vi "Uncompress SEQ line.vi"(4 "error in":errorcluster, 6 "SEQ file refnum":refnum<file>) -> (0 "error out":errorcluster, 2 "Pixel Array":u8[](array[numeric]))   [LabVIEW 2016]
doc: "// *******************************************************************\nBYTE *unCompress( int length, BYTE *buffer )\n{\n BYTE *s,*d, dif;\n WORD pixel;\n\n s = buffer;\n d = full; /* Set up buffer pointers */\n *d++ = *s++; /* Get first pixel */\n length--; /* and adjust counter */\n while (length-- > 0) /* While not EOL */\n {\n pixel = *(WORD *)s++; /* Fetch TWO bytes! */\n // Process the even nibble.\n if ((pixel & 0x0f) == 0x0f)\n { // A nibble of 15 indicates overflow;Next byte contains\n // a new pixel. This byte is on an odd nibble boundary, and mask.\n *d++ = (BYTE)((pixel >> 4) & 0xff); /* Next whole pixel */\n pixel = (WORD)*s++; /* Read next byte */\n length--; /* and adjust counter */\n }\n else\n { // Regular signed nibble difference\n dif = (BYTE)(pixel & 0x0F);\n if (pixel & 0x08)\n *d = (BYTE) (*(d-1) - (dif - 7));\n else\n *d = (BYTE) (*(d-1) + dif);\n d++;\n }\n // Now process the odd nibble.\n if ((pixel & 0xf0) == 0xf0)\n { // A nibble of 15 indicates overflow; Next byte contains a new\n // pixel. This byte is on a byte boundary, so simply fetch it.\n *d++ = *s++; /* Next pixel */\n length--; /* and adjust counter */\n }\n else\n { // Regular signed nibble difference\n dif = (BYTE)((pixel & 0xF0) >>4);\n if (pixel & 0x80)\n *d = (BYTE) (*(d-1) - (dif -7));\n else\n *d = (BYTE) (*(d-1) + dif);\n d++; /* Increment destination */\n }\n }\n return(full);\n}"
panel:
  out "#bytes in\ncompressed\nline":u16(graph)
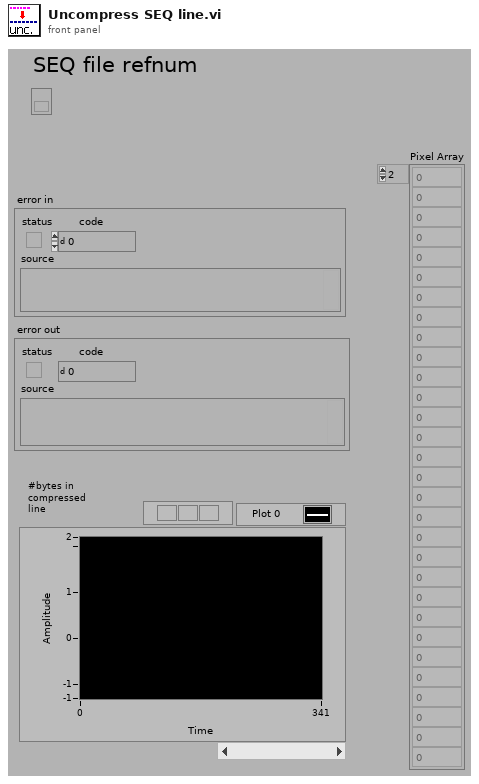
[diagram p1: front panel]
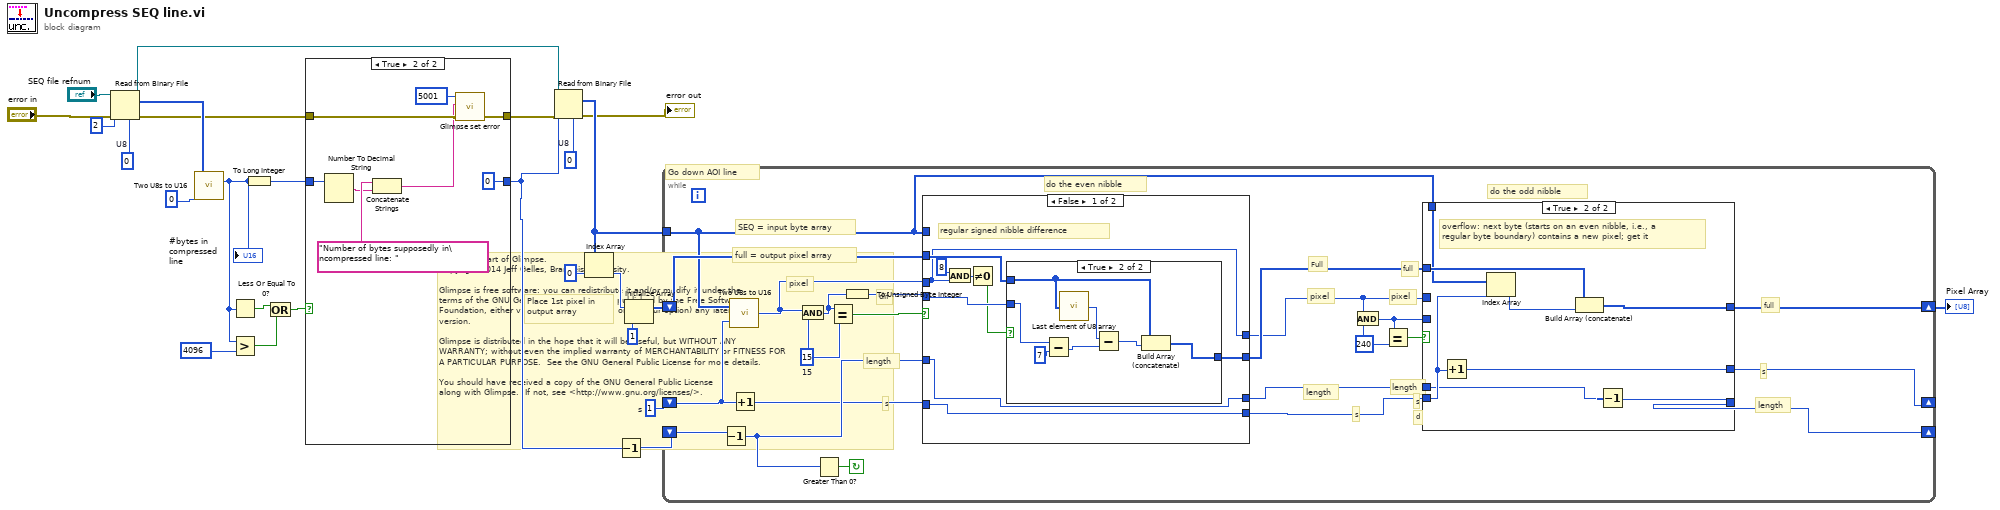
[diagram p0: block diagram]
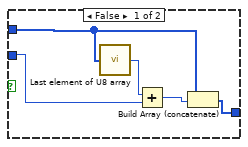
[diagram p3: hidden frame]
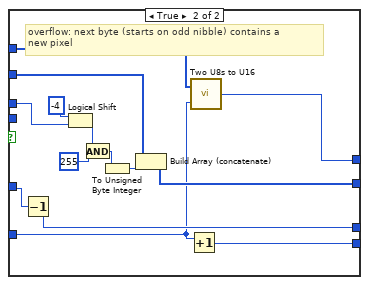
[diagram p4: hidden frame]
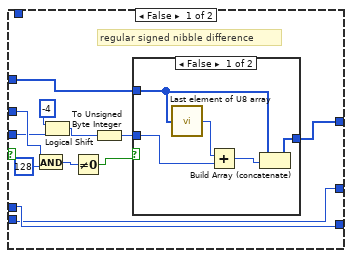
[diagram p5: hidden frame]
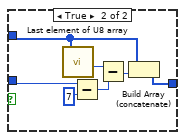
[diagram p6: hidden frame]
diagram:
  w15 = 1  # s
  w18 = u8 0  # U8
  w23 = u8 0  # U8
  # "This file is part of Glimpse. \nCopyright 2014 Jeff Gelles, Brandeis University.    \n\nGlimpse is free software: you can redistribute it and/or modify it under the \nterms of the GNU General Public License as published by the Free Software \nFoundation, either version 3 of the License, or (at your option) any later \nversion.\n\nGlimpse is distributed in the hope that it will be useful, but WITHOUT ANY \nWARRANTY; without even the implied warranty of MERCHANTABILITY or FITNESS FOR \nA PARTICULAR PURPOSE.  See the GNU General Public License for more details.\n\nYou should have received a copy of the GNU General Public License\nalong with Glimpse.  If not, see <http://www.gnu.org/licenses/>."
  # "Place 1st pixel in\noutput array"
  # "Go down AOI line"
  n1 = Read from Binary File(5:w23, 8:"error in", 10:2 ("count"), 11:"SEQ file refnum") -> (0:w2:errorcluster, 2:w19:u8[], 3:w17:refnum<file>)  [unwired: 3 out]
  n2 = call "Two U8s to U16.vi"("Index of first byte"=0 ("index"), "Byte array"=w19) -> ("Output word"=w6:u16)
  "#bytes in\ncompressed\nline" <- w6
  n3 = Less Or Equal To 0?(x=w6) -> (x <= 0?=w9:bool)
  n4 = Greater?(x=w6, y=u16 4096) -> (0:w5:bool)
  n5 = To Long Integer(number=w6) -> (32bit integer=w4:i32)
  n6 = Or(x=w9, y=w5) -> (x .or. y?=w8:bool)
  n7 = case shown="True" w8 {
    tunnel: w4 -> [w28 w32]
    tunnel: [w28 0] -> w3
    tunnel: w2 -> [w27 w34]
    tunnel: [w27 w35] -> w1
    frame False {
    }
    frame True {
      n8 = Number To Decimal String(number=w32) -> (decimal integer string=w30:string)  [unwired: 1 out]
      n9 = Concatenate Strings("Number of bytes supposedly in\ncompressed line: " ("string"), w30) -> (w29:string)
      n10 = call "Glimpse set error.vi"("code"=5001, "Additional information"=w29, "error in"=w34) -> ("error out"=w35:errorcluster)  [unwired: 5 out]
    }
  }
  n11 = Read from Binary File(5:w18, 8:w1, 10:w3, 11:w17) -> (0:→"error out":errorcluster, 2:w16:u8[])  [unwired: 4 out]
  n12 = Index Array(array=w16, index=0) -> (element=w13:u8)
  n13 = Decrement(x=w3) -> (x-1=w26:i32)
  n14 = Initialize Array(w13, 1) -> (w12:u8[])
  n15 = while {
    tunnel: w16 -> [w37]
    shift-left: w12 -> [w52]
    shift-right: [w40] -> w11
    shift-left: w26 -> [w55]
    shift-right: [w38] -> _
    shift-left: w15 -> [w50]
    shift-right: [w39] -> _
    stop <- w53 continue-if-true
    w45 = u8 240 ("15")
    w58 = u8 15  # 15
    # "do the even nibble"
    # "s"
    # "s"
    # "full"
    # "pixel"
    # "d"
    # "s"
    # "length"
    # "full"
    # "length"
    # "do the odd nibble"
    # "pixel"
    # "SEQ = input byte array"
    # "full = output pixel array"
    # "s"
    # "length"
    # "pixel"
    # "length"
    # "Full"
    # "dif"
    n16 = Decrement(x=w55) -> (x-1=w54:i32)
    n17 = call "Two U8s to U16.vi"("Index of first byte"=w50, "Byte array"=w37) -> ("Output word"=w49:u16)
    n18 = Increment(x=w50) -> (x+1=w51:i32)
    n19 = And(x=w49, y=w58) -> (x .and. y?=w56:u16)
    n20 = Greater Than 0?(x=w54) -> (x > 0?=w53:bool)
    n21 = Equal?(x=w56, y=w58) -> (x = y?=w57:bool)
    n22 = To Unsigned Byte Integer(number=w56) -> (unsigned 8bit integer=w48:u8)
    n23 = case shown="False" w57 {
      tunnel: w51 -> [w63 w80]
      tunnel: [w63 w93] -> w41
      tunnel: w49 -> [w59 w85]
      tunnel: w48 -> [w67 _]
      tunnel: [w62 w87] -> w44
      tunnel: w54 -> [w61 w92]
      tunnel: [w61 w91] -> w42
      tunnel: w52 -> [w60 w86]
      tunnel: [w59 w82] -> w43
      tunnel: w37 -> [_ w81]
      frame False {
        # "regular signed nibble difference"
        n24 = And(x=u8 8 ("15"), y=w59) -> (x .and. y?=w66:u16)
        n25 = Not Equal To 0?(x=w66) -> (x != 0?=w64:bool)
        n26 = case shown="True" w64 {
          tunnel: w67 -> [w70 w79]
          tunnel: w60 -> [w69 w75]
          tunnel: [w68 w77] -> w62
          frame False {
            n27 = call "Last element of U8 array.vi"("Array"=w69) -> ("Last element"=w71:u8)
            n28 = Add(x=w71, y=w70) -> (x+y=w72:u8)
            n29 = Build Array (concatenate)(w69, w72) -> (w68:u8[])
          }
          frame True {
            n30 = Subtract(x=w79, y=u8 7) -> (x-y=w74:u8)
            n31 = call "Last element of U8 array.vi"("Array"=w75) -> ("Last element"=w76:u8)
            n32 = Subtract(x=w76, y=w74) -> (x-y=w73:u8)
            n33 = Build Array (concatenate)(w75, w73) -> (w77:u8[])
          }
        }
      }
      frame True {
        # "overflow: next byte (starts on odd nibble) contains a \nnew pixel"
        n34 = Decrement(x=w92) -> (x-1=w91:i32)
        n35 = Logical Shift(y=i16 -4, x=w85) -> (x << y=w89:u16)
        n36 = And(x=w89, y=u8 255) -> (x .and. y?=w84:u16)
        n37 = To Unsigned Byte Integer(number=w84) -> (unsigned 8bit integer=w83:u8)
        n38 = Build Array (concatenate)(w86, w83) -> (w87:u8[])
        n39 = Increment(x=w80) -> (x+1=w93:i32)
        n40 = call "Two U8s to U16.vi"("Index of first byte"=w80, "Byte array"=w81) -> ("Output word"=w82:u16)
      }
    }
    n41 = And(x=w43, y=w45) -> (x .and. y?=w47:u16)
    n42 = Equal?(x=w47, y=w45) -> (x = y?=w46:bool)
    n43 = case shown="True" w46 {
      tunnel: w41 -> [w98 w124]
      tunnel: w44 -> [w99 w119]
      tunnel: [w101 w125] -> w40
      tunnel: [w105 w122] -> w38
      tunnel: w42 -> [w105 w121]
      tunnel: w43 -> [w100 _]
      tunnel: [w98 w123] -> w39
      tunnel: w47 -> [w97 _]
      tunnel: w37 -> [_ w118]
      frame False {
        # "regular signed nibble difference"
        n44 = And(x=w100, y=u8 128) -> (x .and. y?=w95:u16)
        n45 = Logical Shift(y=i16 -4, x=w97) -> (x << y=w102:u16)
        n46 = Not Equal To 0?(x=w95) -> (x != 0?=w94:bool)
        n47 = To Unsigned Byte Integer(number=w102) -> (unsigned 8bit integer=w96:u8)
        n48 = case shown="False" w94 {
          tunnel: w96 -> [w106 w117]
          tunnel: [w108 w112] -> w101
          tunnel: w99 -> [w107 w113]
          frame False {
            n49 = call "Last element of U8 array.vi"("Array"=w107) -> ("Last element"=w110:u8)
            n50 = Add(x=w110, y=w106) -> (x+y=w109:u8)
            n51 = Build Array (concatenate)(w107, w109) -> (w108:u8[])
          }
          frame True {
            n52 = call "Last element of U8 array.vi"("Array"=w113) -> ("Last element"=w115:u8)
            n53 = Subtract(x=w117, y=u8 7) -> (x-y=w114:u8)
            n54 = Subtract(x=w115, y=w114) -> (x-y=w111:u8)
            n55 = Build Array (concatenate)(w113, w111) -> (w112:u8[])
          }
        }
      }
      frame True {
        # "overflow: next byte (starts on an even nibble, i.e., a\nregular byte boundary) contains a new pixel; get it"
        n56 = Increment(x=w124) -> (x+1=w123:i32)
        n57 = Index Array(array=w118, index=w124) -> (element=w120:u8)
        n58 = Build Array (concatenate)(w119, w120) -> (w125:u8[])
        n59 = Decrement(x=w121) -> (x-1=w122:i32)
      }
    }
  }
  "Pixel Array" <- w11
